vi "ShooterPneumatics(SubVI).vi"   [LabVIEW 2017]
uses:
  EnuSqu.ctl
  <vilib>/Rock Robotics/WPI/Solenoid/WPI_SolenoidValue.ctl
  <vilib>/Rock Robotics/WPI/Solenoid/WPI_SolenoidSetEnum.vi
  <vilib>/Rock Robotics/WPI/Utilities/WPI_GetSetVariantRefNum.vi
types:
  T1 = typedef "EnuSqu.ctl" = enum16{"0", "1", "2", "3"}
  T2 = typedef "WPI_SolenoidValue.ctl" = enum16{"Off", "On", "Forward", "Reverse"}
  T3 = typedef "WPI_SolenoidDevRef.ctl" = cluster{"DevStatus":errorcluster, "Pneumatics Control Module":u8, "Forward Solenoid Channel":T4, "Reverse Solenoid Channel":T4}
  T4 = typedef "WPI_SolenoidChannel.ctl" = enum8{"Solenoid 0", "Solenoid 1", "Solenoid 2", "Solenoid 3", "Solenoid 4", "Solenoid 5", "Solenoid 6", "Solenoid 7", "Invalid"}
  T5 = typedef "WPI_RobotDriveDevRef.ctl" = cluster{"DevStatus":errorcluster, "Motors[]":T6[], "Square Inputs":bool, "Max Output":dbl}
  T6 = typedef "WPI_MotorControlDeviceRef.ctl" = cluster{"DeviceStatus":errorcluster, "Type":T7, "PWM":cluster{"PWM Channel":T8, "DeadBand":T9}, "CAN":cluster{"Device Number":u8, "SetOutput VI Ref":variant, "GetOutput VI Ref":variant, "Enable VI Ref":variant, "Disable VI Ref":variant, "Data":variant}, "Invert":bool, "DIO PWM":cluster{"PWM \"Enable\" Channel":T8, "DIOChannel":T10, "PWM Rate":dbl}}
  T7 = typedef "WPI_MotorControlType.ctl" = enum16{"PWM", "CAN", "DIO PWM"}
  T8 = typedef "FPGA_DIOPWMChannel.ctl" = enum8{"PWM 0", "PWM 1", "PWM 2", "PWM 3", "PWM 4", "PWM 5", "PWM 6", "PWM 7", "PWM 8", "PWM 9", "PWM MXP 0", "PWM MXP 1", "PWM MXP 2", "PWM MXP 3", "PWM MXP 4", "PWM MXP 5", "PWM MXP 6", "PWM MXP 7", "PWM MXP 8", "PWM MXP 9", "Invalid"}
  T9 = typedef "WPI_PWMDeadband.ctl" = cluster{"Name":string, "maxPositivePwm":i32, "minPositivePwm":i32, "centerPwm":i32, "maxNegativePwm":i32, "minNegativePwm":i32, "angularRange":u16}
  T10 = typedef "FPGA_DIOChannel.ctl" = enum8{"DIO 0", "DIO 1", "DIO 2", "DIO 3", "DIO 4", "DIO 5", "DIO 6", "DIO 7", "DIO 8", "DIO 9", "DIO MXP 0", "DIO MXP 1", "DIO MXP 2", "DIO MXP 3", "DIO MXP 4", "DIO MXP 5", "DIO MXP 6", "DIO MXP 7", "DIO MXP 8", "DIO MXP 9", "DIO MXP 10", "DIO MXP 11", "DIO MXP 12", "DIO MXP 13", "DIO MXP 14", "DIO MXP 15", "SPI Port CS1", "SPI Port CS2", "SPI Port CS3", "SPI Port MISO", "SPI Port MOSI", "Invalid"}
  T11 = typedef "WPI_JoystickDevRef.ctl" = cluster{"Device":T12}
  T12 = typedef "WPI_JoystickDeviceEnum.ctl" = enum16{"USB 0", "USB 1", "USB 2", "USB 3", "USB 4", "USB 5"}
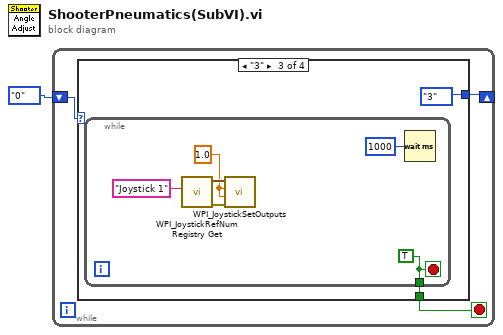
[diagram p0: block diagram]
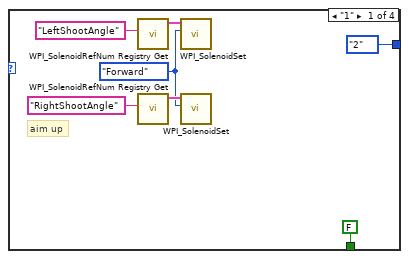
[diagram p2: hidden frame]
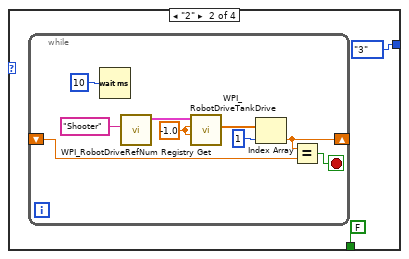
[diagram p3: hidden frame]
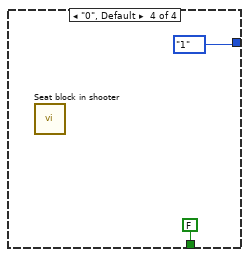
[diagram p4: hidden frame]
diagram:
  n1 = while {
    shift-right: [w3] -> _
    shift-left: EnuSqu."0" -> [w4]
    stop <- w2 stop-if-true
    n2 = case shown="\"3\"" w4 {
      tunnel: [EnuSqu."2" EnuSqu."3" EnuSqu."3" EnuSqu."1"] -> w3
      tunnel: [FALSE FALSE w23 FALSE] -> w2
      frame "1" {
        w7 = WPI_SolenoidValue."Forward" ("Value")
        # "aim up"
        n3 = call <vilib>:"WPI_SolenoidRefNum Registry Get.vi"("refnum name"="LeftShootAngle") -> ("SolenoidDevRef"=w8:T3)  [unwired: 9 in, 1 out]
        n4 = call <vilib>:"WPI_SolenoidRefNum Registry Get.vi"("refnum name"="RightShootAngle") -> ("SolenoidDevRef"=w10:T3)  [unwired: 9 in, 1 out]
        n5 = call-poly <vilib>:"WPI_SolenoidSet.vi"("Value"=w7, "SolenoidDevRef"=w8) -> ()  [unwired: 8 in, 2 out]
        n6 = call-poly <vilib>:"WPI_SolenoidSet.vi"("Value"=w7, "SolenoidDevRef"=w10) -> ()  [unwired: 8 in, 2 out]
      }
      frame "2" {
        n7 = while {
          shift-right: [w17] -> _
          shift-left: _ -> [w16]
          stop <- w14 stop-if-true
          w21 = -1.0
          n8 = Wait (ms)(milliseconds to wait=u32 10) -> ()  [unwired: 1 out]
          n9 = call <vilib>:"WPI_RobotDriveRefNum Registry Get.vi"("refnum name"="Shooter") -> ("RobotDriveDevRef"=w22:T5)  [unwired: 9 in, 1 out]
          n10 = call <vilib>:"WPI_RobotDriveTankDrive.vi"("Right axis value"=w21, "Left axis value"=w21, "RobotDriveDevRef"=w22) -> ("Motor Values"=w19:dbl[])  [unwired: 6 in, 2 out]
          n11 = Index Array(array=w19, index=1) -> (element=w17:dbl)
          n12 = Equal?(x=w17, y=w16) -> (x = y?=w14:bool)
        }
      }
      frame "3" {
        n13 = while {
          tunnel: [w26] -> w23
          stop <- w26 stop-if-true
          w26 = TRUE
          w25 = sgl 1.0 ("Right Rumble")
          n14 = call <vilib>:"WPI_JoystickRefNum Registry Get.vi"("refnum name"="Joystick 1") -> ("error out"=w30:errorcluster, "JoystickDevRef"=w29:T11)  [unwired: 9 in]
          n15 = call <vilib>:"WPI_JoystickSetOutputs.vi"("error in (no error)"=w30, "Right Rumble"=w25, "Left Rumble"=w25, "JoystickDevRef"=w29) -> ()  [unwired: 6 in, 2 out]
          n16 = Wait (ms)(milliseconds to wait=u32 1000) -> ()  [unwired: 1 out]
        }
      }
      frame "0", Default {
        n17 = call "Seat block in shooter.vi"() -> ()  [unwired: 11 in, 1 out]
      }
    }
  }
